vi "Add Enum Property Node.vi"(7 "Node Type":string, 9 "Enum Inputs":T1, 10 "Property Parent":string, 11 "Doc Ref":refnum<k20>) -> (1 "Updated Node Ref":refnum<k20>, 3 "Node Found?":bool)   [LabVIEW 2025]
uses:
  <resource>/objmgr/DOMUserDefRef.rc
  Shared/Types/NodeFilteringOptions.ctl
  Types/TD NodeRef Map Action.ctl
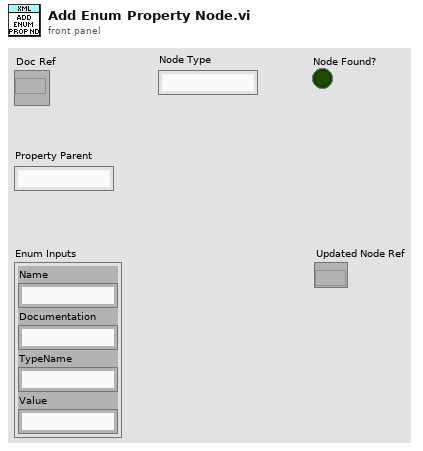
[diagram p1: front panel]
types:
  T1 = cluster{"Name":string, "Documentation":string, "TypeName":string, "Value":string}
  T2 = typedef "NodeFilteringOptions.ctl" = enum16{"GetCustomDeviceNode", "GetAllChannelNodes", "GetAllSectionNodes", "GetAllWaveformNodes", "GetFirstChannelNode", "GetFirstSectionNode", "GetFirstWaveformNode", "GetSpecificSectionNode", "GetSpecificCustomDeviceNode", "GetSpecificChannelNode", "GetSpecificWaveformNode", "GetMatchedNamedNode", "GetEnumDefinitionsNode", "GetSpecificEnumDefinitionNode", "GetAllEnumDefinitionNodes", "GetDynamicChannelNodes"}
  T3 = typedef "TD NodeRef Map Action.ctl" = enum16{"Init", "Add XMLNodeRef", "Delete XMLNodeRef", "Add TDNodeRefs", "Delete TDNodeRefs", "Clear TDNodeRefs", "Add ChildXMLNodeRef", "Delete ChildXMLNodeRef", "Get All Keys", "Update ParentName", "Get", "skip"}
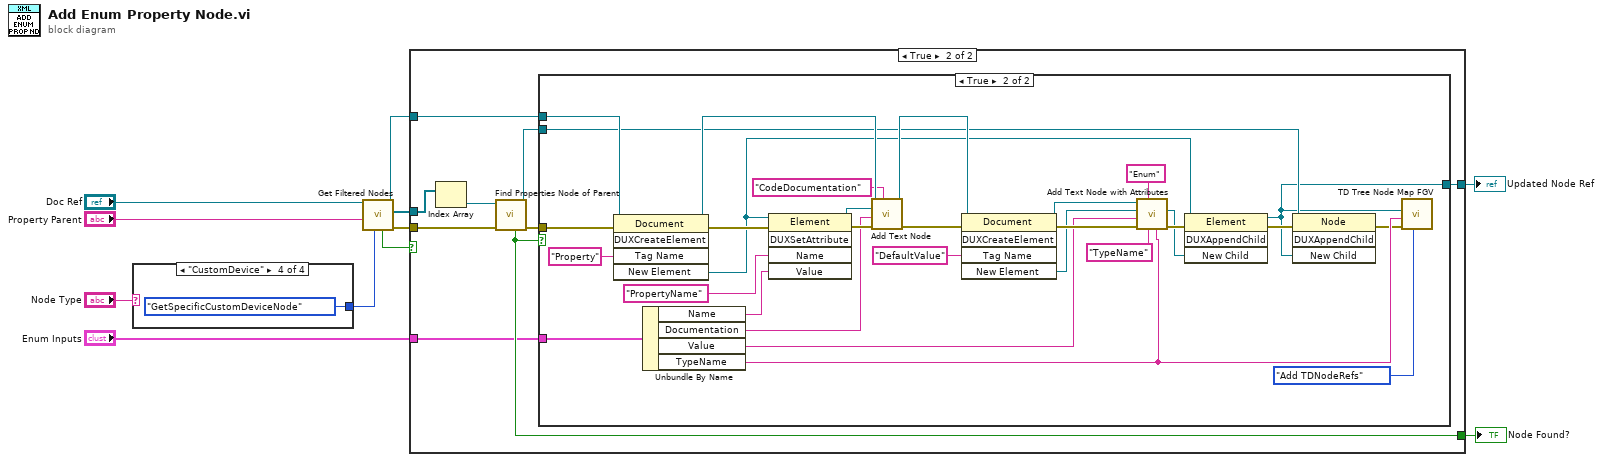
[diagram p0: block diagram]
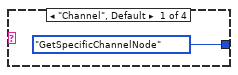
[diagram p4: hidden frame]
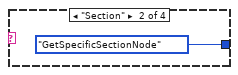
[diagram p5: hidden frame]
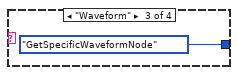
[diagram p6: hidden frame]
diagram:
  n1 = case shown="\"CustomDevice\"" "Node Type" {
    tunnel: [NodeFilteringOptions."GetSpecificChannelNode" ("Node Filtering") NodeFilteringOptions."GetSpecificSectionNode" ("Node Filtering") NodeFilteringOptions."GetSpecificWaveformNode" ("Node Filtering") NodeFilteringOptions."GetSpecificCustomDeviceNode" ("Node Filtering")] -> w9
    frame "Channel", Default {
    }
    frame "Section" {
    }
    frame "Waveform" {
    }
    frame "CustomDevice" {
    }
  }
  n2 = call "Get Filtered Nodes.vi"("Node Filtering"=w9, "Node Name"="Property Parent", "Document in"="Doc Ref") -> ("error out"=w7:errorcluster, "Filtered Nodes"=w4:refnum<k20>[], "Document out"=w6:refnum<k20>, "Node Found?"=w5:bool)  [unwired: 4 in, 1 out]
  n3 = case shown="True" w5 {
    tunnel: [_ w22] -> w11
    tunnel: w7 -> [_ w21]
    tunnel: w6 -> [_ w20]
    tunnel: w4 -> [_ w19]
    tunnel: "Enum Inputs" -> [_ w17]
    tunnel: [_ w16] -> w1
    frame False {
    }
    frame True {
      n4 = Index Array(array=w19) -> (element=w18:refnum<k20>)  [unwired: 1 in]
      n5 = call "Find Properties Node of Parent.vi"("error in"=w21, "Node"=w18) -> ("error out"=w23:errorcluster, "Poperties Node"=w24:refnum<k20>, "Node Found?"=w22:bool)  [unwired: 7 in]
      n6 = case shown="True" w22 {
        tunnel: w24 -> [_ w37]
        tunnel: w23 -> [_ w44]
        tunnel: w20 -> [_ w43]
        tunnel: w17 -> [_ w42]
        tunnel: [_ w25] -> w16
        frame False {
        }
        frame True {
          n7 = invoke class="Document" method="DUXCreateElement"(reference=w43, error in=w44, "Tag Name"="Property") -> (reference out=w50:refnum<k20>, error out=w54:errorcluster, "New Element"=w38:refnum<k20>)  [unwired: 2 in, 2 out]
          n8 = Unbundle By Name(w42) -> ("Name"=w41:string, "Documentation"=w40:string, "Value"=w29:string, "TypeName"=w28:string)
          n9 = invoke class="Element" method="DUXSetAttribute"(reference=w38, error in=w54, "Name"="PropertyName", "Value"=w41) -> (reference out=w49:refnum<k20>, error out=w53:errorcluster)  [unwired: 1 in, 3 out]
          n10 = call "Add Text Node.vi"("Tag Name"="CodeDocumentation", "error in"=w53, "Tag Data"=w40, "Element in"=w49, "Document in"=w50) -> ("error out"=w46:errorcluster, "Document out"=w48:refnum<k20>)  [unwired: 4 in, 1 out]
          n11 = invoke class="Document" method="DUXCreateElement"(reference=w48, error in=w46, "Tag Name"="DefaultValue") -> (reference out=w34:refnum<k20>, error out=w36:errorcluster, "New Element"=w35:refnum<k20>)  [unwired: 2 in, 2 out]
          n12 = call "Add Text Node with Attributes.vi"("Attr Value"=w28, "Attr Name"="TypeName", "Tag Name"="Enum" ("Tag Data"), "error in"=w36, "Tag Data"=w29, "Element in"=w35, "Document in"=w34) -> ("error out"=w33:errorcluster, "Element out"=w32:refnum<k20>)  [unwired: 2 in, 1 out]
          n13 = invoke class="Element" method="DUXAppendChild"(reference=w38, error in=w33, "New Child"=w32) -> (reference out=w25:refnum<k20>, error out=w39:errorcluster)  [unwired: 1 in, 2 out]
          n14 = invoke class="Node" method="DUXAppendChild"(reference=w37, error in=w39, "New Child"=w25) -> (error out=w26:errorcluster)  [unwired: 1 in, 3 out]
          n15 = call "TD Tree Node Map FGV.vi"("Action"=TD_NodeRef_Map_Action."Add TDNodeRefs", "error in"=w26, "Node Name"=w28, "Attribute Node"=w25) -> ()  [unwired: 2 in, 6 out]
        }
      }
    }
  }
  "Node Found?" <- w11
  "Updated Node Ref" <- w1
